vi "Joystick FIX.vi"() -> ()   [LabVIEW 2023]
uses:
  <vilib>/Analysis/coordinate.llb/Angle Units.ctl
  <vilib>/Analysis/coordinate.llb/Angle Range (Degree).ctl
  <vilib>/Analysis/coordinate.llb/Wrap Angle (scalar).vi
  <vilib>/Analysis/NI_AAL_Angle.lvlib
panel:
  out "XY after\nDEADBAND":cluster{"X":dbl, "Y":dbl}={"X"=1.0, "Y"=0.04}
  in  "resting steer angle (deg)":dbl=90.0 format="%#_13g"
  in  "Jy input":dbl=0.04 min=-1.0 max=1.0 format="%.4f"
  in  "Jx input":dbl=1.0 min=-1.0 max=1.0 format="%.4f"
  in  "Jr input":dbl=1.0 min=-1.0 max=1.0 format="%.4f"
  out "Jr":dbl=1.0 format="%#.4f"
  in  "Reset\nFILTER":bool
  in  "Max dx/dt":dbl=10.0
  in  "apply\nFILTER":bool
  out "error out":errorcluster
  in  "error in (no error)":errorcluster
  in  "axis dead band":dbl=0.05000000000000004 format="%#_13g"
  out "Jx":dbl=0.9992009587217894 format="%#.4f"
  out "Jy":dbl format="%#.4f"
  out "theta (deg)":dbl=2.29061004263853
  out "theta (rad)":dbl=0.039978687123290044
  out "R":dbl=1.0
  out "Joystick":cluster{dbl[], dbl[]}(graph)={[0.0, 1.0], [0.0, 0.04]}
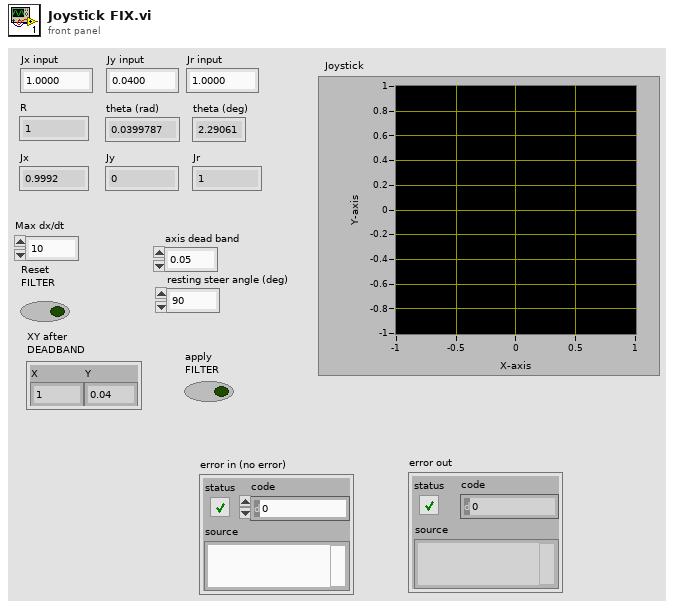
[diagram p1: front panel]
types:
  T1 = typedef "NI_AAL_Angle.lvlib/Angle Range (Degree).ctl" = u16
  T2 = typedef "NI_AAL_Angle.lvlib/Angle Units.ctl" = i32
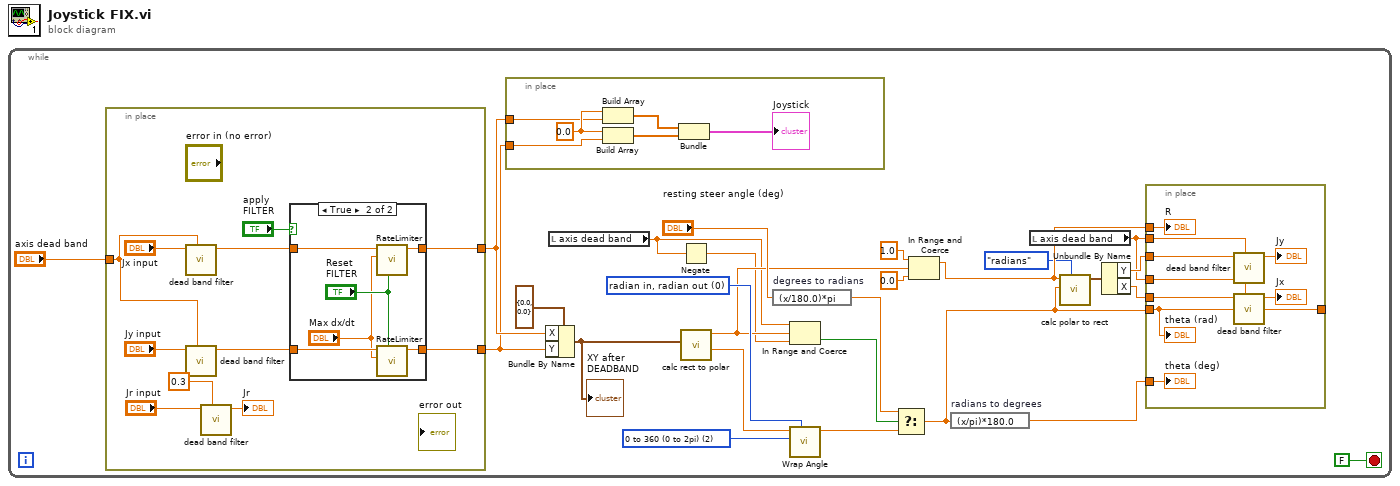
[diagram p0: block diagram]
diagram:
  n1 = while {
    stop <- FALSE stop-if-true
    w14 = T1 2 items=["none", "-180 to 180 (-pi to pi)", "0 to 360 (0 to 2pi)"] ("angle range")
    w15 = T2 0 items=["radian in, radian out", "radian in, degree out", "degree in, degree out", "degree in, radian out"] ("angle units")
    n2 = in-place {
      in-place-border: [w34] -> w21
      in-place-border: [w33] -> w20
      in-place-border: "axis dead band" -> [w31]
      n3 = call "dead band filter.vi"("deadband"=w31, "input"="Jx input") -> ("output"=w35:dbl)  [unwired: 9 in]
      n4 = call "dead band filter.vi"("deadband"=w31, "input"="Jy input") -> ("output"=w32:dbl)  [unwired: 9 in]
      n5 = call "dead band filter.vi"("deadband"=0.3, "input"="Jr input") -> ("output"=→"Jr":dbl)  [unwired: 9 in]
      n6 = case shown="True" "apply\nFILTER" {
        tunnel: w35 -> [w38 w45]
        tunnel: [w38 w44] -> w34
        tunnel: [w39 w43] -> w33
        tunnel: w32 -> [w39 w42]
        frame False {
        }
        frame True {
          n7 = call "RateLimiter.vi"("Reset"="Reset\nFILTER", "Max dx/dt"="Max dx/dt", "Input"=w45) -> ("Output"=w44:dbl)  [unwired: 8 in]
          n8 = call "RateLimiter.vi"("Reset"="Reset\nFILTER", "Max dx/dt"="Max dx/dt", "Input"=w42) -> ("Output"=w43:dbl)  [unwired: 8 in]
        }
      }
    }
    n9 = in-place {
      in-place-border: w21 -> [w59]
      in-place-border: w20 -> [w58]
      w60 = 0.0 ("element")
      n10 = Build Array(w60, w59) -> (w56:dbl[])
      n11 = Build Array(w60, w58) -> (w55:dbl[])
      n12 = Bundle(w56, w55) -> (→"Joystick":cluster{dbl[], dbl[]})  [unwired: 1 in]
    }
    n13 = Bundle By Name(cluster=cluster{"X":dbl, "Y":dbl} {"X"=0.0, "Y"=0.0} ("XY"), "X"=w21, "Y"=w20) -> (w8:cluster{"X":dbl, "Y":dbl})
    "XY after\nDEADBAND" <- w8
    n14 = local read "axis dead band"() -> (w4:dbl)
    n15 = Negate(x=w4) -> (-x=w3:dbl)
    n16 = call "calc rect to polar.vi"("XY"=w8) -> ("angle (rad)"=w10:dbl, "Magnitude"=w11:dbl)  [unwired: 8 in, 1 out]
    n17 = expression code="(x/180.0)*pi" "degrees to radians"("resting steer angle (deg)") -> (w5:dbl)
    n18 = In Range and Coerce(upper limit=w4, x=w11, lower limit=w3) -> (In Range?=w12:bool)  [unwired: 1 out]
    n19 = call-poly <vilib>:"Wrap Angle.vi"("angle units"=w15, "angle range"=w14, "angle in"=w10) -> ("angle out"=w7:dbl)  [unwired: 7 in, 1 out]
    n20 = Select(t=w5, s=w12, f=w7) -> (s? t:f=w23:dbl)
    n21 = In Range and Coerce(upper limit=1.0, x=w11, lower limit=0.0 ("x")) -> (coerced(x)=w22:dbl)  [unwired: 1 out]
    n22 = expression code="(x/pi)*180.0" "radians to degrees"(w23) -> (w24:dbl)
    n23 = local read "axis dead band"() -> (w2:dbl)
    n24 = call "calc polar to rect.vi"("units"=enum16{"degrees", "radians"}."radians", "angle"=w23, "mag"=w22) -> ("XY"=w16:cluster{"X":dbl, "Y":dbl})  [unwired: 8 in]
    n25 = Unbundle By Name(w16) -> ("Y"=w25:dbl, "X"=w26:dbl)
    n26 = in-place {
      in-place-border: w26 -> [w52]
      in-place-border: w25 -> [w50]
      in-place-border: w24 -> [w54]
      in-place-border: w23 -> [w48]
      in-place-border: w22 -> [w53]
      in-place-border: [w48] -> _
      in-place-border: w2 -> [w47]
      in-place-border: w2 -> [w46]
      n27 = call "dead band filter.vi"("deadband"=w47, "input"=w50) -> ("output"=→"Jy":dbl)  [unwired: 9 in]
      n28 = call "dead band filter.vi"("deadband"=w46, "input"=w52) -> ("output"=→"Jx":dbl)  [unwired: 9 in]
      "theta (deg)" <- w54
      "theta (rad)" <- w48
      "R" <- w53
    }
  }
